vi "Get Sub Exports.vi"(0 "NSIS_Installer in":refnum<class "Compound_Installer.lvclass">, 5 "Sub Installer Name":string, 11 "error in (no error)":errorcluster) -> (4 "NSIS_Installer out":refnum<class "Compound_Installer.lvclass">, 6 "Export":refnum<class "Export.lvclass">, 10 "found":bool, 15 "error out":errorcluster)   [LabVIEW 2017, in "CL_G3_VIComponentBuilder.lvlib" / "Compound_Installer.lvclass"]
doc: "Gets a sub installer (aka export) by its unique name."
uses:
  Compound_Installer.lvclass
  Exports/Export.lvclass
  Compound_Installer.lvclass/Compound_Installer.ctl
  Accessors/Read Sub Exports.vi
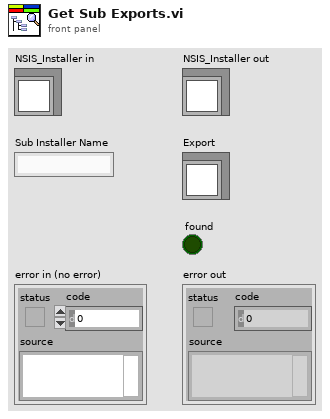
[diagram p1: front panel]
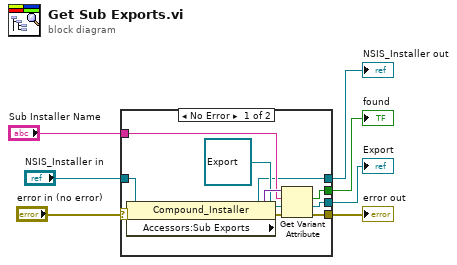
[diagram p0: block diagram]
diagram:
  n1 = case shown="No Error" "error in (no error)" {
    selector: "error in (no error)" -> [w11 w19]
    tunnel: [w10 w19] -> w6
    tunnel: [w13 w18] -> w4
    tunnel: "NSIS_Installer in" -> [w16 w18]
    tunnel: "Sub Installer Name" -> [w14 _]
    tunnel: [w9 _] -> w2
    tunnel: [w8 _] -> w1
    frame No Error {
      n2 = property class="Compound_Installer"(reference=w16, error in=w11) -> (reference out=w13:refnum<class "Compound_Installer.lvclass">, error out=w12:errorcluster, "Accessors:Sub Exports"=w17:variant)
      n3 = Get Variant Attribute(Variant=w17, name=w14, default value (empty Variant)=refnum<class "Export.lvclass"> refnum ("CL_G3_VIComponentBuilder.lvlib:Export"), error in=w12) -> (found=w8:bool, value=w9:refnum<class "Export.lvclass">, error out=w10:errorcluster)  [unwired: 1 out]
    }
    frame Error {
    }
  }
  "error out" <- w6
  "NSIS_Installer out" <- w4
  "Export" <- w2
  "found" <- w1
